vi "Pre Launch Init.vi"(11 "PLCHandler in":refnum<class "PLCHandler.lvclass">) -> (0 "error out":errorcluster, 3 "PLCHandler out":refnum<class "PLCHandler.lvclass">)   [LabVIEW 2022 SP3, in "PLCHandler.lvlib" / "PLCHandler.lvclass"]
doc: "(<B>Filename</B>: Actor Framework.lvlib:Actor.lvclass:Pre Launch Init.vi)\n\nDefines behavior that occurs after the Launch Actor method is invoked but before the actor's Actor Core method begins running.\n\nThe Pre Launch Init method is guaranteed to finish before the Launch Actor method returns to its caller and before the actor itself receives any messages. Any references that the Pre Launch Init method obtains are guaranteed to have the same lifetime as the actor itself. Any errors that the Pre Launch Init method returns will abort the launch.\n\nBy default, this method does nothing. A descendant class may override it to define behavior."
uses:
  PLCHandler.lvclass
  Typedefs/PLC Settings.ctl
  PLCHandler.lvclass/PLCHandler.ctl
  <vilib>/ActorFramework/Actor/Actor.lvclass
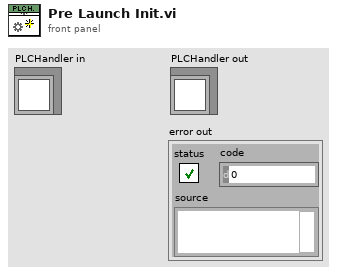
[diagram p1: front panel]
types:
  T1 = typedef "PLC Settings.ctl" = cluster{"Port":refnum<visa-resource-name>, "BaudRate":u32, "Wakeup Signal Address ":u16, "Acquisiton Address":u16, "Acknowledgement Address":u16, "Sleep Address":u32}
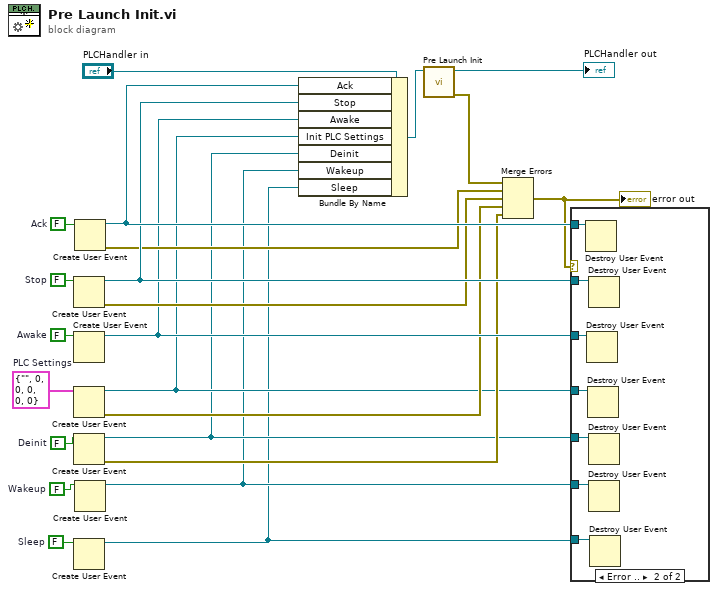
[diagram p0: block diagram]
diagram:
  w4 = FALSE  # Sleep
  w5 = FALSE  # Wakeup
  w10 = FALSE  # Deinit
  w11 = T1 {"Port"="", "BaudRate"=0, "Wakeup Signal Address "=0, "Acquisiton Address"=0, "Acknowledgement Address"=0, "Sleep Address"=0}  # PLC Settings
  w13 = FALSE  # Awake
  w21 = FALSE  # Stop
  w22 = FALSE  # Ack
  n1 = Create User Event(user event datatype=w21) -> (user event=w17:refnum<user-event>, error out=w15:errorcluster)  [unwired: 1 in]
  n2 = Create User Event(user event datatype=w13) -> (user event=w12:refnum<user-event>)  [unwired: 1 in, 1 out]
  n3 = Create User Event(user event datatype=w11) -> (user event=w7:refnum<user-event>, error out=w8:errorcluster)  [unwired: 1 in]
  n4 = Create User Event(user event datatype=w10) -> (user event=w6:refnum<user-event>, error out=w9:errorcluster)  [unwired: 1 in]
  n5 = Create User Event(user event datatype=w4) -> (user event=w1:refnum<user-event>)  [unwired: 1 in, 1 out]
  n6 = Create User Event(user event datatype=w22) -> (user event=w18:refnum<user-event>, error out=w16:errorcluster)  [unwired: 1 in]
  n7 = Create User Event(user event datatype=w5) -> (user event=w2:refnum<user-event>)  [unwired: 1 in, 1 out]
  n8 = Bundle By Name(cluster="PLCHandler in", "Ack"=w18, "Stop"=w17, "Awake"=w12, "Init PLC Settings"=w7, "Deinit"=w6, "Wakeup"=w2, "Sleep"=w1) -> (w20:refnum<class "PLCHandler.lvclass">)
  n9 = call-parent "Pre Launch Init.vi"("Actor in"=w20) -> ("error out"=w3:errorcluster, "Actor out"=→"PLCHandler out":refnum<class "PLCHandler.lvclass">)  [unwired: 9 in]
  n10 = Merge Errors(w3, w16, w15, w8, w9) -> (w14:errorcluster)
  "error out" <- w14
  n11 = case shown="Error .." w14 {
    tunnel: w18 -> [_ w30]
    tunnel: w17 -> [_ w29]
    tunnel: w12 -> [_ w28]
    tunnel: w6 -> [_ w27]
    tunnel: w7 -> [_ w26]
    tunnel: w2 -> [_ w25]
    tunnel: w1 -> [_ w24]
    frame No Error {
    }
    frame Error {
      n12 = Destroy User Event(user event=w30) -> ()  [unwired: 1 in, 1 out]
      n13 = Destroy User Event(user event=w28) -> ()  [unwired: 1 in, 1 out]
      n14 = Destroy User Event(user event=w26) -> ()  [unwired: 1 in, 1 out]
      n15 = Destroy User Event(user event=w29) -> ()  [unwired: 1 in, 1 out]
      n16 = Destroy User Event(user event=w27) -> ()  [unwired: 1 in, 1 out]
      n17 = Destroy User Event(user event=w25) -> ()  [unwired: 1 in, 1 out]
      n18 = Destroy User Event(user event=w24) -> ()  [unwired: 1 in, 1 out]
    }
  }
